vi "duf file read.vi"(8 "error in (no error)":errorcluster, 10 "NEW PARAMETERS":T1, 11 "Main Ref":T2) -> (0 "error out":errorcluster, 2 "output cluster":T1, 3 "Main Ref 2":T2)   [LabVIEW 2025]
panel:
  in  "Fuel Description :":string
  in  "Batch Ref Number :":string
  in  "Date and Time :":string
  out "text":string
  out "Tested Date":string
  out "Tested By :-":string
  out "Operator :":string
  out "XY Graph":cluster{"X":dbl[], "Y":dbl[]}[](graph)
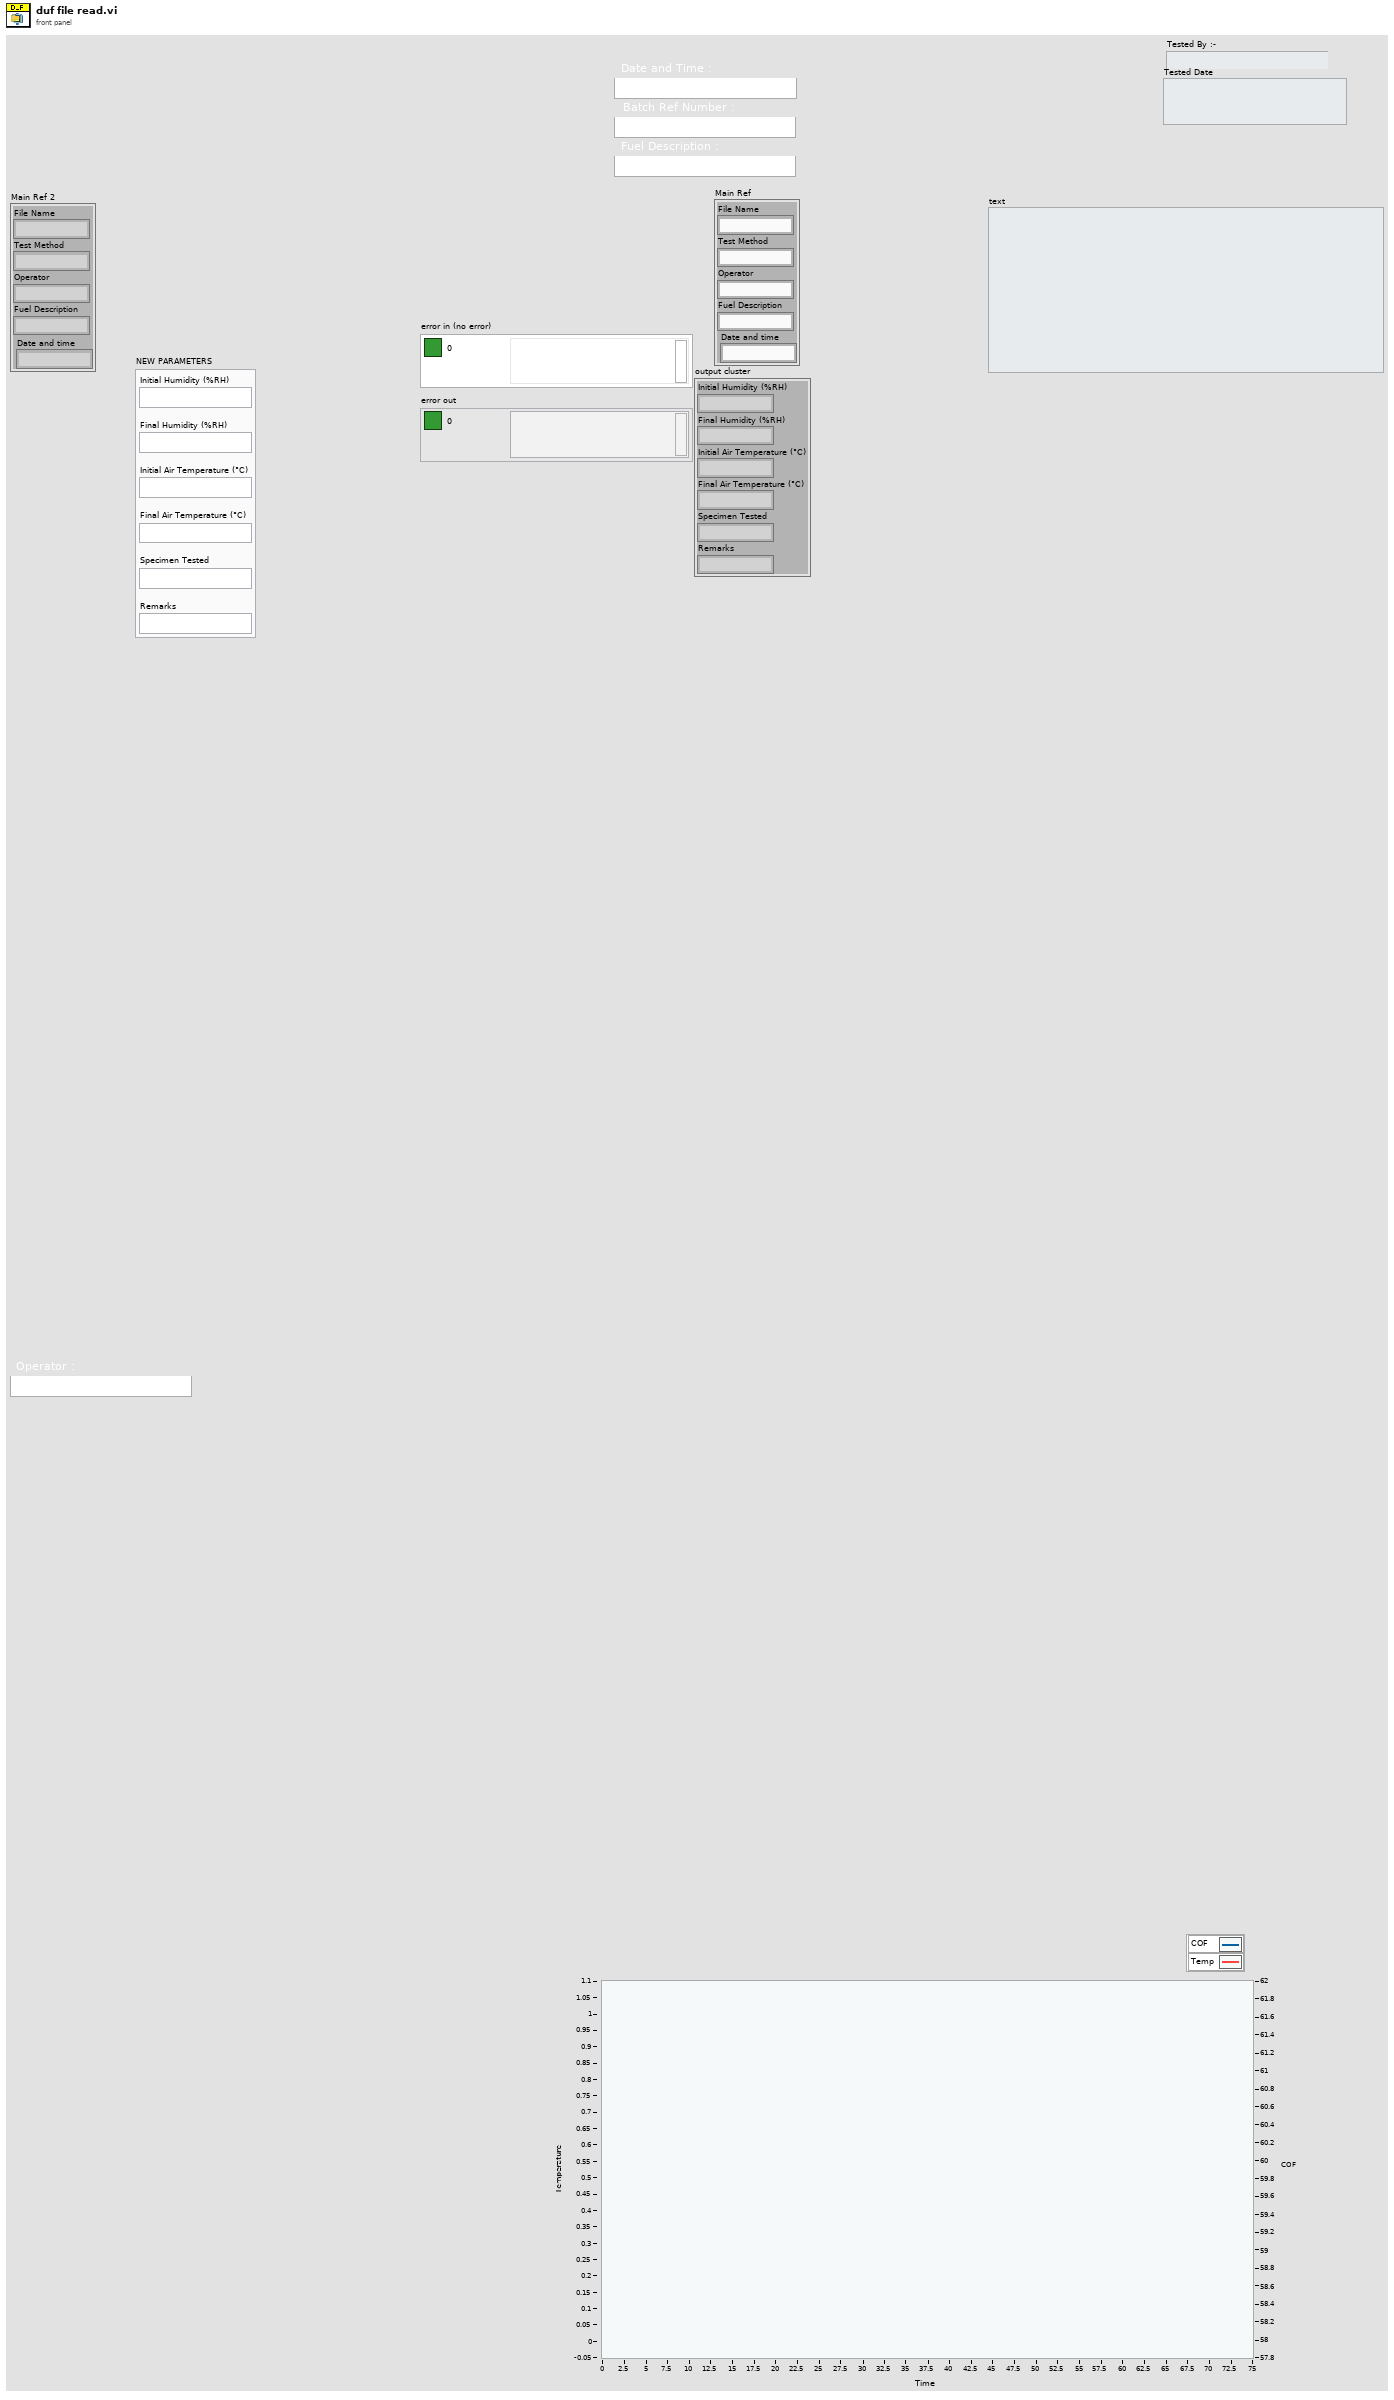
[diagram p1: front panel]
types:
  T1 = cluster{"Initial Humidity (%RH)":string, "Final Humidity (%RH)":string, "Initial Air Temperature (°C)":string, "Final Air Temperature (°C)":string, "Specimen Tested":string, "Remarks":string}
  T2 = cluster{"File Name":string, "Test Method":string, "Operator":string, "Fuel Description":string, "Date and time":string}
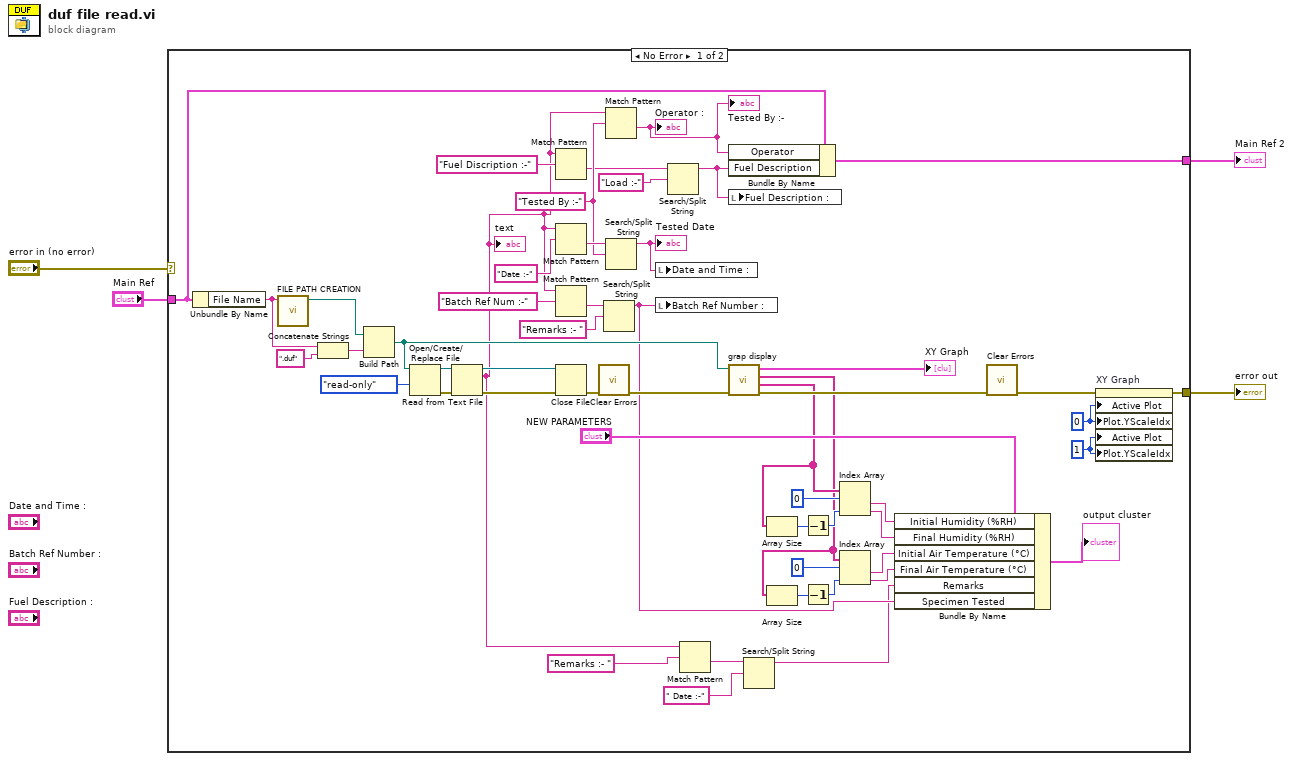
[diagram p0: block diagram]
diagram:
  n1 = case shown="No Error" "error in (no error)" {
    tunnel: "Main Ref" -> [w27 w57]
    tunnel: [w30 _] -> w3
    tunnel: [w26 w57] -> w1
    frame No Error {
      w43 = u32 1 ("Active Plot")
      w44 = u32 0 ("Active Plot")
      w49 = "Tested By :-" ("regular expression")
      n2 = Unbundle By Name(w27) -> ("File Name"=w32:string)
      n3 = call "FILE PATH CREATION.vi"("FILE NAME :"=w32) -> ("FILE OUT"=w34:path)  [unwired: 9 in, 1 out]
      n4 = Concatenate Strings(w32, ".duf" ("Substring")) -> (w35:string)
      n5 = Build Path(base path=w34, name or relative path=w35) -> (appended path=w31:path)
      n6 = Open/Create/Replace File(file path (use dialog)=w31, access (0:read/write)=enum16{"read/write", "read-only", "write-only"}."read-only") -> (refnum out=w54:refnum<file>, error out=w55:errorcluster)  [unwired: 4 in, 1 out]
      n7 = Read from Text File(file (use dialog)=w54, error in=w55) -> (refnum out=w52:refnum<file>, text=w9:string, error out=w53:errorcluster)  [unwired: 2 in, 1 out]
      "text" <- w9
      n8 = Match Pattern(string=w9, regular expression="Fuel Discription :-") -> (after substring=w37:string)  [unwired: 1 in, 3 out]
      n9 = Match Pattern(string=w9, regular expression="Date :-") -> (after substring=w50:string)  [unwired: 1 in, 3 out]
      n10 = Match Pattern(string=w9, regular expression="Batch Ref Num :-") -> (after substring=w38:string)  [unwired: 1 in, 3 out]
      n11 = Close File(refnum=w52, error in=w53) -> (error out=w42:errorcluster)  [unwired: 1 out]
      n12 = call <vilib>:"Clear Errors.vi"("error in (no error)"=w42) -> ("error out"=w41:errorcluster)  [unwired: 5 in, 1 out]
      n13 = Search/Split String(string=w38, search string/char (-)="Remarks :- ") -> (substring before match=w10:string)  [unwired: 1 in, 2 out]
      n14 = Match Pattern(string=w9, regular expression=w49) -> (after substring=w29:string)  [unwired: 1 in, 3 out]
      "Tested By :-" <- w29
      "Operator :" <- w29
      n15 = Search/Split String(string=w50, search string/char (-)=w49) -> (substring before match=w48:string)  [unwired: 1 in, 2 out]
      "Tested Date" <- w48
      n16 = local write "Date and Time :"(w48) -> ()
      n17 = local write "Batch Ref Number :"(w10) -> ()
      n18 = Search/Split String(string=w37, search string/char (-)="Load :-") -> (substring before match=w28:string)  [unwired: 1 in, 2 out]
      n19 = Match Pattern(string=w9, regular expression="Remarks :- " ("search string/char (-)")) -> (after substring=w7:string)  [unwired: 1 in, 3 out]
      n20 = Bundle By Name(cluster=w27, "Operator"=w29, "Fuel Description"=w28) -> (w26:T2)
      n21 = local write "Fuel Description :"(w28) -> ()
      n22 = call "grap display.vi"("error in"=w41, "file path (dialog if empty)"=w31) -> ("error out"=w46:errorcluster, "HUMIDITY"=w15:string[], "AIR TEMPERATURE"=w14:string[], "XY GRAPH"=→"XY Graph":cluster{"X":dbl[], "Y":dbl[]}[])  [unwired: 6 in]
      n23 = Search/Split String(string=w7, search string/char (-)=" Date :-") -> (substring before match=w5:string)  [unwired: 1 in, 2 out]
      n24 = Array Size(array=w15) -> (size(s)=w16:i32)
      n25 = Array Size(array=w14) -> (size(s)=w23:i32)
      n26 = Decrement(x=w16) -> (x-1=w17:i32)
      n27 = Decrement(x=w23) -> (x-1=w22:i32)
      n28 = Index Array(array=w15, index #1=0 ("index"), index #2=w17) -> (element #1=w13:string, element #2=w12:string)
      n29 = Index Array(array=w14, index #1=0 ("index"), index #2=w22) -> (element #1=w20:string, element #2=w19:string)
      n30 = Bundle By Name(cluster="NEW PARAMETERS", "Initial Humidity (%RH)"=w13, "Final Humidity (%RH)"=w12, "Initial Air Temperature (°C)"=w20, "Final Air Temperature (°C)"=w19, "Remarks"=w5, "Specimen Tested"=w10) -> (→"output cluster":T1)
      n31 = call <vilib>:"Clear Errors.vi"("error in (no error)"=w46) -> ("error out"=w45:errorcluster)  [unwired: 5 in, 1 out]
      n32 = property on="XY Graph" class="XYGraph (strict)"(error in=w45, "Active Plot"=w44, "Plot.YScaleIdx"=w44, "Active Plot"=w43, "Plot.YScaleIdx"=w43) -> (error out=w30:errorcluster)  [unwired: 1 in, 1 out]
    }
    frame Error {
    }
  }
  "error out" <- w3
  "Main Ref 2" <- w1
